vi "Handle Error.vi"(8 "error in (no error)":errorcluster, 11 "Controller in":refnum<class "Controller.lvclass">) -> (0 "error out":errorcluster, 2 "stop actor?":bool=TRUE, 3 "Controller out":refnum<class "Controller.lvclass">)   [LabVIEW 2016, in "Controller.lvlib" / "Controller.lvclass"]
doc: "(<B>Filename</B>: Actor Framework.lvlib:Actor.lvclass:Handle Error.vi)\n\nDefines how the actor handles an error that occurred while processing a message. By default, this method does nothing except stop the actor."
uses:
  Controller.lvclass
  <vilib>/ActorFramework/Actor/Actor.lvclass
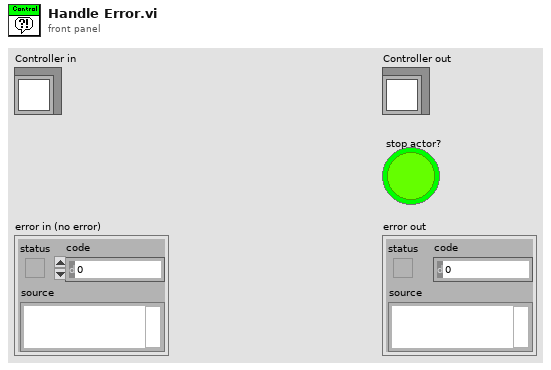
[diagram p1: front panel]
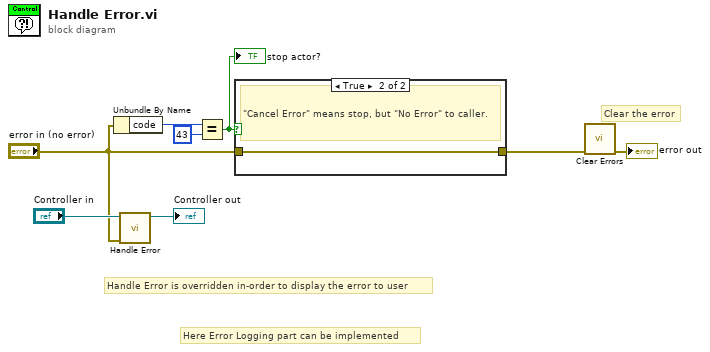
[diagram p0: block diagram]
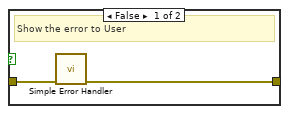
[diagram p2: hidden frame]
diagram:
  # "Here Error Logging part can be implemented"
  # "Clear the error"
  # "Handle Error is overridden in-order to display the error to user"
  n1 = Unbundle By Name("error in (no error)") -> ("code"=w3:i32)
  n2 = call-parent "Handle Error.vi"("error in (no error)"="error in (no error)", "Actor in"="Controller in") -> ("Actor out"=→"Controller out":refnum<class "Controller.lvclass">)  [unwired: 7 in, 2 out]
  n3 = Equal?(x=w3, y=43) -> (x = y?=w1:bool)
  "stop actor?" <- w1
  n4 = case shown="True" w1 {
    tunnel: [w10 w11] -> w6
    tunnel: "error in (no error)" -> [w9 w11]
    frame False {
      # "Show the error to User"
      n5 = call <vilib>:"Simple Error Handler.vi"("error in (no error)"=w9) -> ("error out"=w10:errorcluster)  [unwired: 4 in, 4 out]
    }
    frame True {
      # "\"Cancel Error\" means stop, but \"No Error\" to caller."
    }
  }
  n6 = call <vilib>:"Clear Errors.vi"("error in (no error)"=w6) -> ("error out"=→"error out":errorcluster)  [unwired: 5 in, 1 out]
